vi "Rate_Limit.vi"(9 "Reset":bool, 10 "Ramp_Rate":dbl, 11 "Input":dbl) -> (3 "Output":dbl)   [LabVIEW 2016, in "ArgosLib.lvlib"]
uses:
  ArgosLib.lvlib
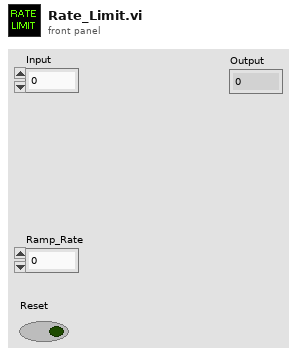
[diagram p1: front panel]
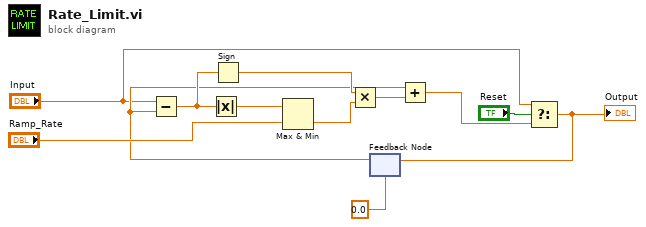
[diagram p0: block diagram]
diagram:
  n1 = feedback #1(0.0) -> (w5:dbl)
  n2 = Subtract(x="Input", y=w5) -> (x-y=w9:dbl)
  n3 = Absolute Value(x=w9) -> (abs(x)=w11:dbl)
  n4 = Sign(1:w9) -> (0:w8:dbl)
  n5 = Max & Min(x=w11, y="Ramp_Rate") -> (min(x,y)=w7:dbl)  [unwired: 1 out]
  n6 = Multiply(x=w8, y=w7) -> (x*y=w6:dbl)
  n7 = Add(x=w5, y=w6) -> (x+y=w2:dbl)
  n8 = Select(t="Input", s="Reset", f=w2) -> (s? t:f=w1:dbl)
  "Output" <- w1
  n9 = feedback-in #1(w1) -> ()
